vi "Main.vi"(8 "error in (no error)":errorcluster, 11 "Process in":refnum<class "TCP Process.lvclass">) -> (0 "error out":errorcluster, 3 "Process out":refnum<class "TCP Process.lvclass">)   [LabVIEW 2019, in "TimingDRV Engine.lvlib" / "TCP Process.lvclass"]
uses:
  TCP Process.lvclass
  C:/Users/nitest/Desktop/CD Project Tools/Source/Engine/Parent Classes/Process/Process.lvclass
  TCP Process.lvclass/TCP Process.ctl
  Parent Classes/Process/Process.lvclass
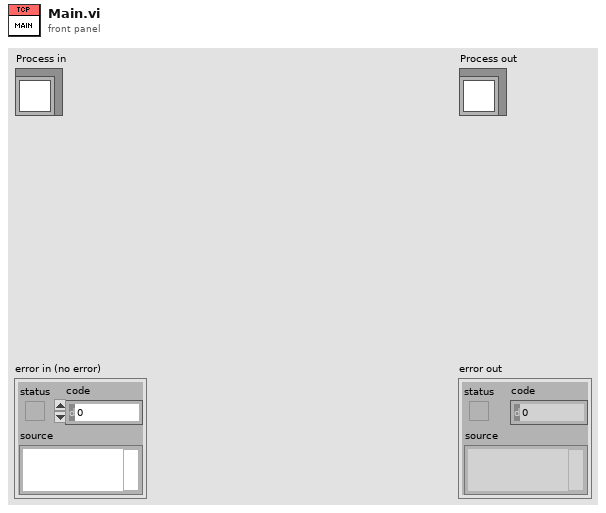
[diagram p1: front panel]
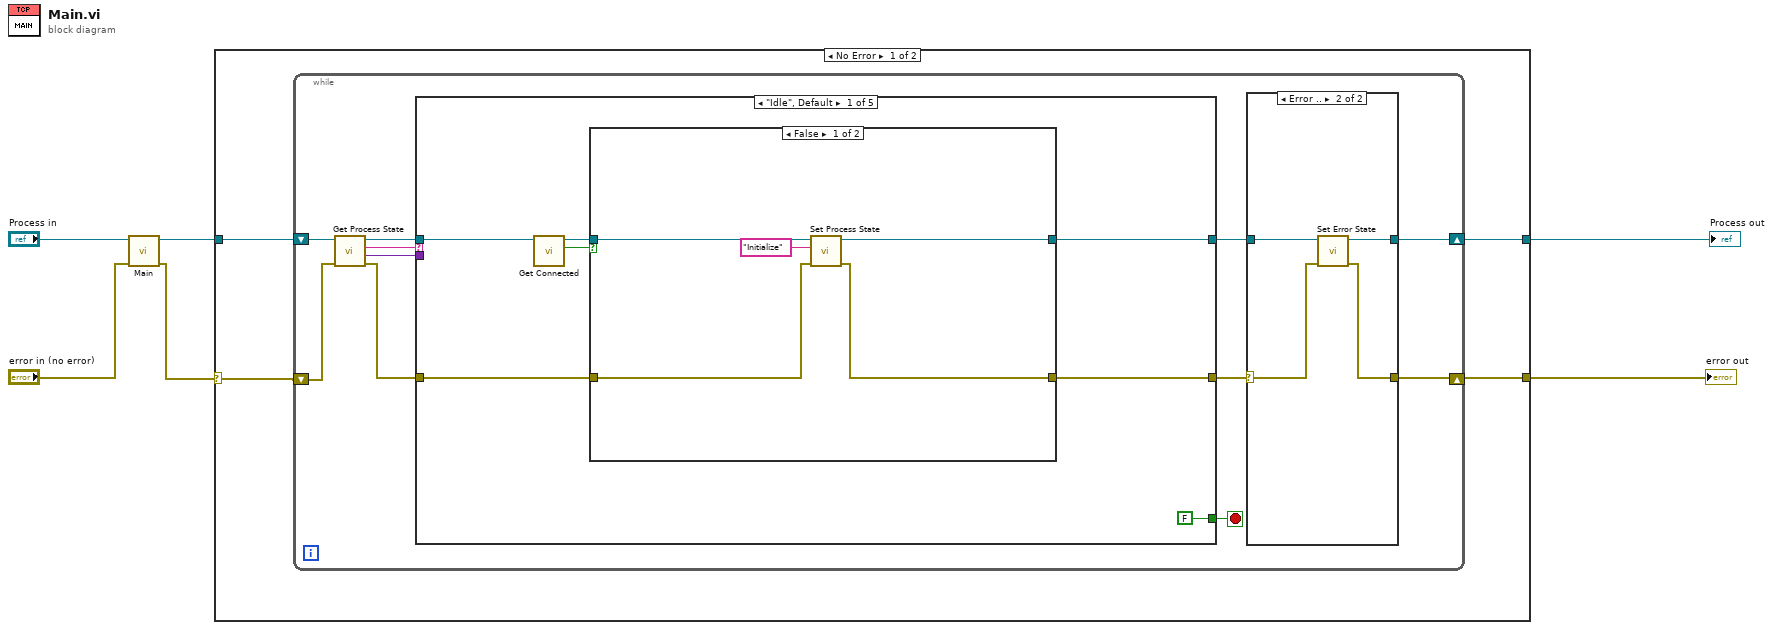
[diagram p0: block diagram]
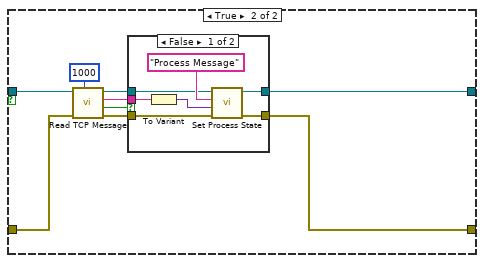
[diagram p3: hidden frame]
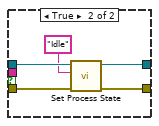
[diagram p4: hidden frame]
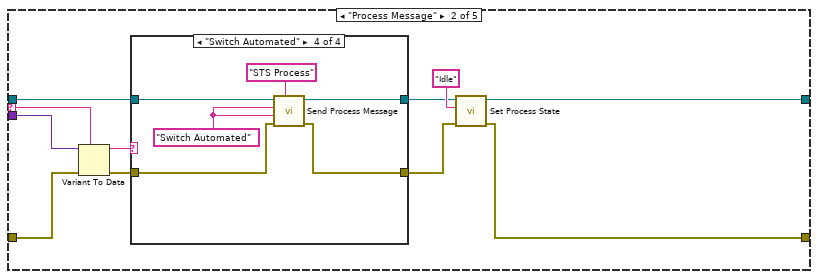
[diagram p5: hidden frame]
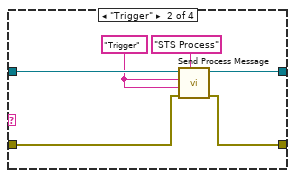
[diagram p7: hidden frame]
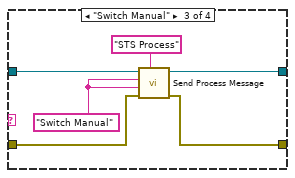
[diagram p8: hidden frame]
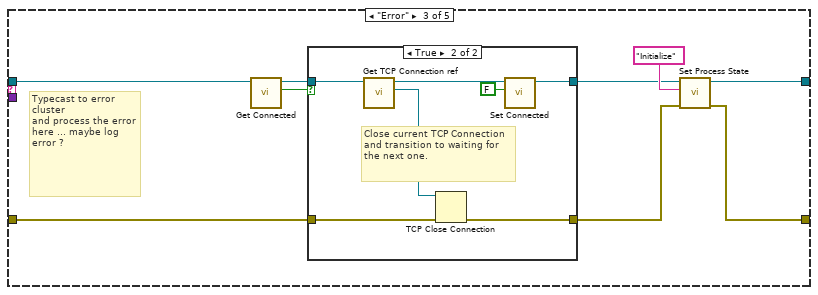
[diagram p9: hidden frame]
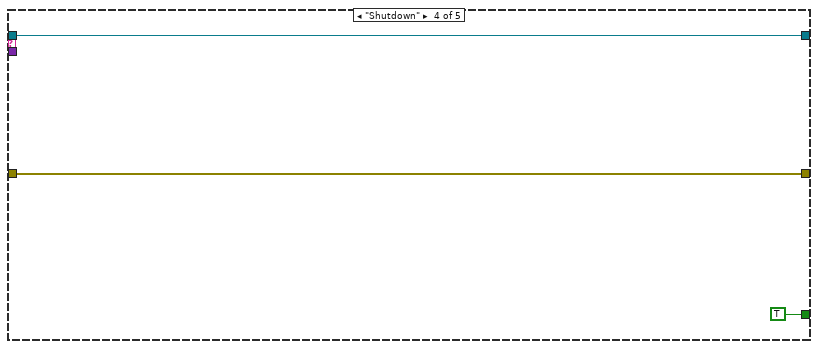
[diagram p11: hidden frame]
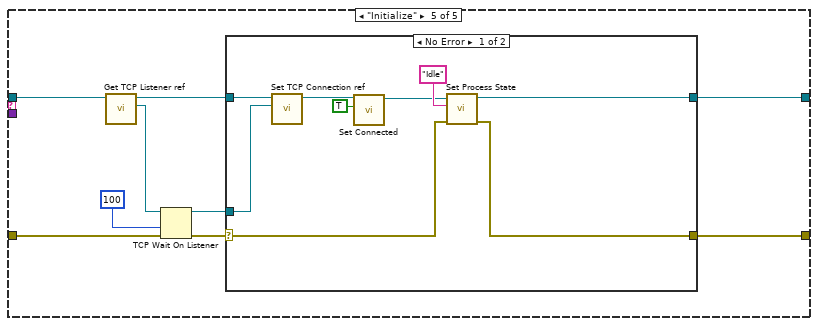
[diagram p12: hidden frame]
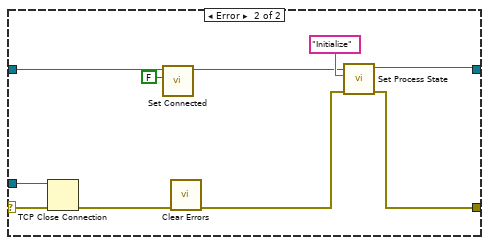
[diagram p13: hidden frame]
diagram:
  n1 = call-parent "Main.vi"("error in (no error)"="error in (no error)", "Process in"="Process in") -> ("error out"=w1:errorcluster, "Process out"=w4:refnum<class "TCP Process.lvclass">)  [unwired: 8 in]
  n2 = case shown="No Error" w1 {
    selector: w1 -> [w7 w141]
    tunnel: w4 -> [w10 w142]
    tunnel: [w9 w142] -> w3
    tunnel: [w8 w141] -> w2
    frame No Error {
      n3 = while {
        shift-right: [w13] -> w9
        shift-left: w10 -> [w20]
        shift-right: [w12] -> w8
        shift-left: w7 -> [w21]
        stop <- w11 stop-if-true
        n4 = call "Get Process State.vi"("error in (no error)"=w21, "Process in"=w20) -> ("error out"=w16:errorcluster, "Payload"=w17:variant, "Command"=w18:string, "Process out"=w19:refnum<class "TCP Process.lvclass">)  [unwired: 6 in]
        n5 = case shown="\"Idle\", Default" w18 {
          selector: w18 -> [_ w70 _ _ _]
          tunnel: w19 -> [w28 w63 w97 w111 w119]
          tunnel: w17 -> [_ w71 _ _ _]
          tunnel: w16 -> [w33 w69 w93 w110 w113]
          tunnel: [w32 w67 w99 w111 w121] -> w15
          tunnel: [w31 w68 w98 w110 w120] -> w14
          tunnel: [FALSE _ _ TRUE _] -> w11
          frame "Idle", Default {
            n6 = call "Get Connected.vi"("TCP Process in"=w28) -> ("Connected"=w29:bool, "TCP Process out"=w30:refnum<class "TCP Process.lvclass">)  [unwired: 9 in]
            n7 = case shown="False" w29 {
              tunnel: w30 -> [w38 w48]
              tunnel: w33 -> [w36 w47]
              tunnel: [w37 w45] -> w32
              tunnel: [w35 w44] -> w31
              frame False {
                n8 = call "Set Process State.vi"("error in (no error)"=w36, "Command"="Initialize", "Process in"=w38) -> ("error out"=w35:errorcluster, "Process out"=w37:refnum<class "TCP Process.lvclass">)  [unwired: 7 in]
              }
              frame True {
                n9 = call "Read TCP Message.vi"("Timeout ms (100)"=1000 ("timeout ms (100)"), "error in (no error)"=w47, "TCP Process in"=w48) -> ("error out"=w40:errorcluster, "Timed out?"=w42:bool, "data out"=w41:string, "TCP Process out"=w46:refnum<class "TCP Process.lvclass">)  [unwired: 5 in]
                n10 = case shown="False" w42 {
                  tunnel: w46 -> [w53 w60]
                  tunnel: w40 -> [w54 w59]
                  tunnel: [w52 w57] -> w45
                  tunnel: [w51 w56] -> w44
                  tunnel: w41 -> [w50 _]
                  frame False {
                    n11 = To Variant(anything=w50) -> (Variant=w49:variant)
                    n12 = call "Set Process State.vi"("error in (no error)"=w54, "Payload"=w49, "Command"="Process Message", "Process in"=w53) -> ("error out"=w51:errorcluster, "Process out"=w52:refnum<class "TCP Process.lvclass">)  [unwired: 6 in]
                  }
                  frame True {
                    n13 = call "Set Process State.vi"("error in (no error)"=w59, "Command"="Idle", "Process in"=w60) -> ("error out"=w56:errorcluster, "Process out"=w57:refnum<class "TCP Process.lvclass">)  [unwired: 7 in]
                  }
                }
              }
            }
          }
          frame "Process Message" {
            n14 = Variant To Data(error in=w69, type=w70, Variant=w71) -> (data=w65:string, error out=w64:errorcluster)
            n15 = case shown="\"Switch Automated\"" w65 {
              tunnel: w64 -> [w73 w76 w82 w88]
              tunnel: w63 -> [w72 w79 w85 w91]
              tunnel: [w72 w78 w84 w90] -> w62
              tunnel: [w73 w75 w81 w87] -> w61
              frame "False", Default {
              }
              frame "Trigger" {
                w74 = "Trigger" ("Command")
                n16 = call "Send Process Message.vi"("Process ID"="STS Process", "error in (no error)"=w76, "Payload"=w74, "Command"=w74, "Process in"=w79) -> ("error out"=w75:errorcluster, "Process out"=w78:refnum<class "TCP Process.lvclass">)  [unwired: 5 in]
              }
              frame "Switch Manual" {
                w80 = "Switch Manual" ("Command")
                n17 = call "Send Process Message.vi"("Process ID"="STS Process", "error in (no error)"=w82, "Payload"=w80, "Command"=w80, "Process in"=w85) -> ("error out"=w81:errorcluster, "Process out"=w84:refnum<class "TCP Process.lvclass">)  [unwired: 5 in]
              }
              frame "Switch Automated" {
                w86 = "Switch Automated" ("Command")
                n18 = call "Send Process Message.vi"("Process ID"="STS Process", "error in (no error)"=w88, "Payload"=w86, "Command"=w86, "Process in"=w91) -> ("error out"=w87:errorcluster, "Process out"=w90:refnum<class "TCP Process.lvclass">)  [unwired: 5 in]
              }
            }
            n19 = call "Set Process State.vi"("error in (no error)"=w61, "Command"="Idle", "Process in"=w62) -> ("error out"=w68:errorcluster, "Process out"=w67:refnum<class "TCP Process.lvclass">)  [unwired: 7 in]
          }
          frame "Error" {
            # "Typecast to error cluster \nand process the error here ... maybe log error ?"
            n20 = call "Get Connected.vi"("TCP Process in"=w97) -> ("Connected"=w96:bool, "TCP Process out"=w95:refnum<class "TCP Process.lvclass">)  [unwired: 9 in]
            n21 = case shown="True" w96 {
              tunnel: w95 -> [w102 w105]
              tunnel: [w102 w108] -> w94
              tunnel: w93 -> [w101 w107]
              tunnel: [w101 w106] -> w92
              frame False {
              }
              frame True {
                # "Close current TCP Connection and transition to waiting for the next one."
                n22 = call "Get TCP Connection ref.vi"("TCP Process in"=w105) -> ("TCP Connection ref"=w103:refnum<k5>, "TCP Process out"=w104:refnum<class "TCP Process.lvclass">)  [unwired: 9 in]
                n23 = TCP Close Connection(connection ID=w103, error in (no error)=w107) -> (error out=w106:errorcluster)  [unwired: 1 in, 1 out]
                n24 = call "Set Connected.vi"("Connected"=FALSE, "TCP Process in"=w104) -> ("TCP Process out"=w108:refnum<class "TCP Process.lvclass">)  [unwired: 9 in]
              }
            }
            n25 = call "Set Process State.vi"("error in (no error)"=w92, "Command"="Initialize", "Process in"=w94) -> ("error out"=w98:errorcluster, "Process out"=w99:refnum<class "TCP Process.lvclass">)  [unwired: 7 in]
          }
          frame "Shutdown" {
          }
          frame "Initialize" {
            n26 = call "Get TCP Listener ref.vi"("TCP Process in"=w119) -> ("Connection ref"=w117:refnum<k5>, "TCP Process out"=w116:refnum<class "TCP Process.lvclass">)  [unwired: 9 in]
            n27 = TCP Wait On Listener(8:w113, 9:100 ("timeout ms (25000)"), 11:w117) -> (0:w115:errorcluster, 4:w114:refnum<k5>)  [unwired: 1 in, 3 out]
            n28 = case shown="No Error" w115 {
              selector: w115 -> [w125 w132]
              tunnel: [w130 w136] -> w121
              tunnel: [w129 w134] -> w120
              tunnel: w116 -> [w127 w139]
              tunnel: w114 -> [w126 w133]
              frame No Error {
                n29 = call "Set TCP Connection ref.vi"("TCP Connection ref"=w126, "TCP Process in"=w127) -> ("TCP Process out"=w124:refnum<class "TCP Process.lvclass">)  [unwired: 9 in]
                n30 = call "Set Connected.vi"("Connected"=TRUE, "TCP Process in"=w124) -> ("TCP Process out"=w123:refnum<class "TCP Process.lvclass">)  [unwired: 9 in]
                n31 = call "Set Process State.vi"("error in (no error)"=w125, "Command"="Idle", "Process in"=w123) -> ("error out"=w129:errorcluster, "Process out"=w130:refnum<class "TCP Process.lvclass">)  [unwired: 7 in]
              }
              frame Error {
                n32 = TCP Close Connection(connection ID=w133, error in (no error)=w132) -> (error out=w131:errorcluster)  [unwired: 1 in, 1 out]
                n33 = call "Set Connected.vi"("Connected"=FALSE, "TCP Process in"=w139) -> ("TCP Process out"=w137:refnum<class "TCP Process.lvclass">)  [unwired: 9 in]
                n34 = call <vilib>:"Clear Errors.vi"("error in (no error)"=w131) -> ("error out"=w135:errorcluster)  [unwired: 5 in, 1 out]
                n35 = call "Set Process State.vi"("error in (no error)"=w135, "Command"="Initialize", "Process in"=w137) -> ("error out"=w134:errorcluster, "Process out"=w136:refnum<class "TCP Process.lvclass">)  [unwired: 7 in]
              }
            }
          }
        }
        n36 = case shown="Error .." w14 {
          selector: w14 -> [w22 w27]
          tunnel: w15 -> [w23 w26]
          tunnel: [w23 w25] -> w13
          tunnel: [w22 w24] -> w12
          frame No Error {
          }
          frame Error {
            n37 = call "Set Error State.vi"("error in (no error)"=w27, "Process in"=w26) -> ("error out"=w24:errorcluster, "Process out"=w25:refnum<class "TCP Process.lvclass">)  [unwired: 8 in]
          }
        }
      }
    }
    frame Error {
    }
  }
  "error out" <- w2
  "Process out" <- w3
